vi "_LO_PAMP_set.vi"(9 "PAV配列":cluster{"VD":dbl, "VG ":dbl, "文字列":string}[](array[cluster]) {"VG" min=0.0 max=2.5; "VD" min=0.0 max=2.5}, 11 "Bias_LO_equip":T1={"Node address"=19, "CAN Interface"="CAN0", "Cartridge band"=10, "Slave Node in"={"Address"=19, "Serial Number"=[16, 71, 55, 76, 1, 8, 0, -15]}, "ObjHandle out"=89653312, "POL"=0, "sb"=1, "GPIB_SM (SIS S,V)"="24", "GPIB_DMM (SIS I)"="22", "GPIB_SM (MAG I) "="25", "GPIB_SG(LO)"="19", "GPIB_PW (PAMP) "="6", "GPIB_TMP1(8ch)"="12", "GPIB_TMP2(2ch)  "="13", "WCA_avg"=10, "Rsen"=10.0, "BiasModule"=1, "LOModule "=1, "WCA_LO_FREQ_SET"={"YTO Low freq. [GHz]"=14.42, "YTO High freq. [GHz]"=17.7, "Kvco"=1, "Lock Pol."=0, "SET LO FREQ"=72.5, "Multiplier"=6.0, "YTO (HEX)"=0, "YTO coarse( FREQ)"=25.0, "NULL PLL INTEGRATOR"=FALSE}, "Res for"=0} {"Res for" items=["none", "series res", "parallel res"]; "WCA_LO_FREQ_SET"."YTO coarse( FREQ)" min=25 max=150 step=0.0001 format="%.3f"; "WCA_LO_FREQ_SET"."Multiplier" min=3 max=6 step=3; "WCA_LO_FREQ_SET"."SET LO FREQ" min=25 max=150 step=0.0001 format="%.3f"; "WCA_LO_FREQ_SET"."Lock Pol." items=["Lower", "Upper"]; "WCA_LO_FREQ_SET"."Kvco" items=["7.5MHz/V", "15MHz/V"]; "WCA_LO_FREQ_SET"."YTO High freq. [GHz]" format="%.3f"; "WCA_LO_FREQ_SET"."YTO Low freq. [GHz]" format="%.3f"; "LOModule" items=["Manual Gunn+PAMP", "B10Lab LO", "WCA LO", "", "YIG発信器"]; "BiasModule" items=["B10Lab Bias", "WCA BiasModule"]; "Slave Node in"."Serial Number" format="%.0x"; "Slave Node in"."Address" format="%.0x"; "Cartridge band" max=10 step=1; "Node address" format="%.0x"}) -> ()   [LabVIEW 2017]
panel:
  in  "WCA_PA_SET":T2={"PA_A_DRAIN_V"=1.0, "PA_A_GATE_V"=0.0, "PA_B_DRAIN_V"=0.0, "PA_B_GATE_V"=0.0} {"PA_B_DRAIN_V" min=0.0 max=2.5; "PA_A_DRAIN_V" min=0.0 max=2.5}
  # "LO freq. [GHz]"
  # "YTO LOW\n/High Freq."
  # "ZERO Intgrtr"
  # "Node Address"
  # "Serial Number"
  # "Drain V"
  # "Gate V"
  # "PA_A (Pol1)"
  # "PA_B (Pol0)"
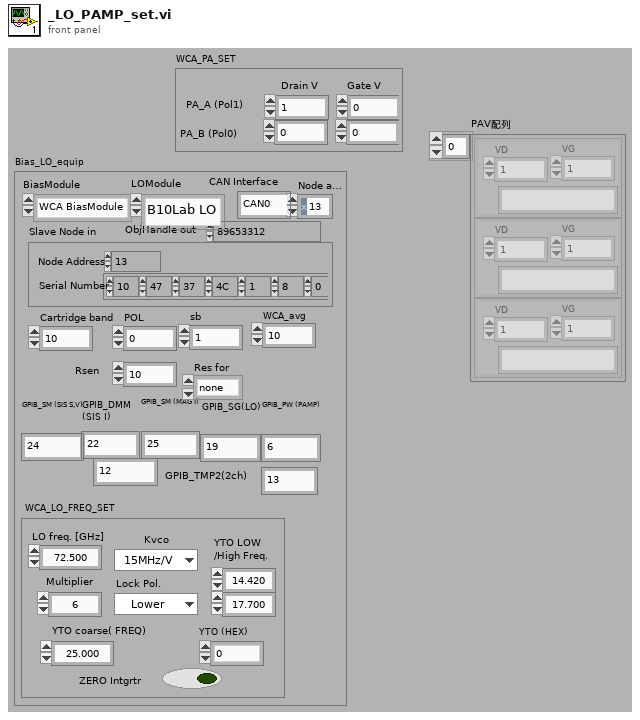
[diagram p1: front panel]
types:
  T1 = cluster{"Node address":u16, "CAN Interface":string, "Cartridge band":u32, "Slave Node in":cluster{"Address":i16, "Serial Number":i8[]}, "ObjHandle out":u32, "POL":u32, "sb":u32, "GPIB_SM (SIS S,V)":string, "GPIB_DMM (SIS I)":string, "GPIB_SM (MAG I) ":string, "GPIB_SG(LO)":string, "GPIB_PW (PAMP) ":string, "GPIB_TMP1(8ch)":string, "GPIB_TMP2(2ch)  ":string, "WCA_avg":i32, "Rsen":dbl, "BiasModule":u16, "LOModule ":u16, "WCA_LO_FREQ_SET":cluster{"YTO Low freq. [GHz]":sgl, "YTO High freq. [GHz]":sgl, "Kvco":u16, "Lock Pol.":u16, "SET LO FREQ":sgl, "Multiplier":sgl, "YTO (HEX)":u16, "YTO coarse( FREQ)":sgl, "NULL PLL INTEGRATOR":bool}, "Res for":u16}
  T2 = cluster{"PA_A_DRAIN_V":dbl, "PA_A_GATE_V":dbl, "PA_B_DRAIN_V":dbl, "PA_B_GATE_V":dbl}
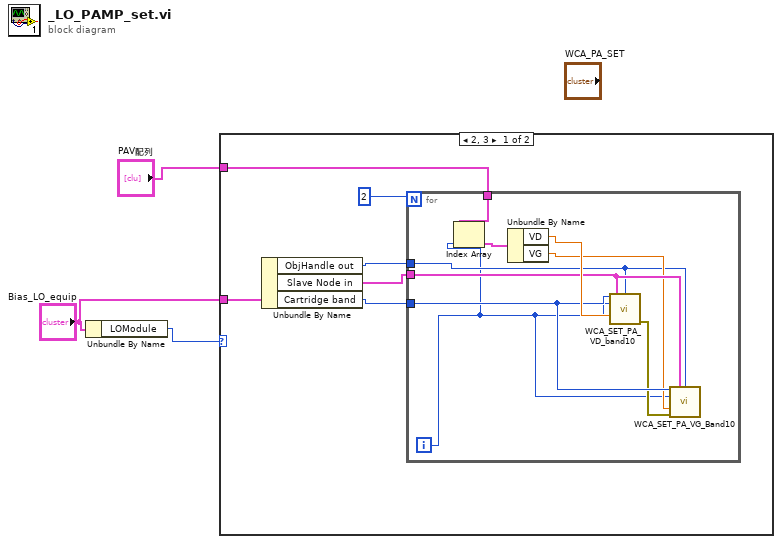
[diagram p0: block diagram]
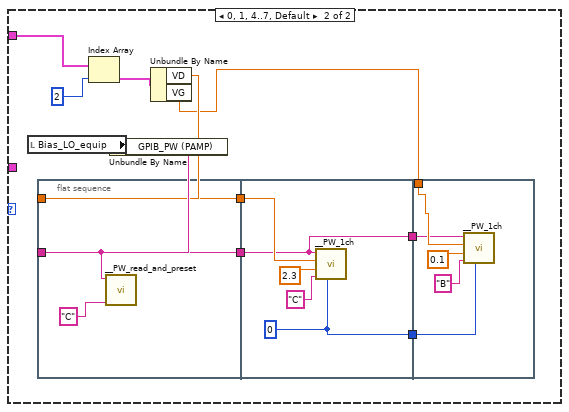
[diagram p2: hidden frame]
diagram:
  n1 = Unbundle By Name("Bias_LO_equip") -> ("LOModule"=w3:u16)
  n2 = case shown="2, 3" w3 {
    tunnel: "PAV配列" -> [w9 w29]
    tunnel: "Bias_LO_equip" -> [w8 _]
    frame 2, 3 {
      n3 = Unbundle By Name(w8) -> ("ObjHandle out"=w5:u32, "Slave Node in"=w7:cluster{"Address":i16, "Serial Number":i8[]}, "Cartridge band"=w6:u32)
      n4 = for {
        N: 2 -> [_]
        tunnel: w9 -> [w17]
        tunnel: w7 -> [w15]
        tunnel: w6 -> [w14]
        tunnel: w5 -> [w12]
        i -> [w10]
        n5 = Index Array(array=w17, index=w10) -> (element=w18:cluster{"VD":dbl, "VG ":dbl, "文字列":string})
        n6 = Unbundle By Name(w18) -> ("VD"=w16:dbl, "VG"=w13:dbl)
        n7 = call "WCA_SET_PA_VD_band10.vi"("Cartridge Band"=w14, "Slave Node in"=w15, "ObjHandle in"=w12, "POL（P0、P1）"=w10, "SET_PA_VD"=w16) -> ("error out"=w11:errorcluster)  [unwired: 9 in, 1 out]
        n8 = call "WCA_SET_PA_VG_Band10.vi"("Cartridge Band"=w14, "Slave Node in"=w15, "ObjHandle in"=w12, "POL（P0、P1）"=w10, "SET_PA_VG"=w13, "error in (no error)"=w11) -> ()  [unwired: 8 in, 2 out]
      }
    }
    frame 0, 1, 4..7, Default {
      n9 = local read "Bias_LO_equip"() -> (w26:T1)
      n10 = flat-sequence {
        tunnel: w24 -> [w32]
        tunnel: w25 -> [w31]
        tunnel: [w31] -> w21
        tunnel: [w32] -> w20
        tunnel: [w34] -> w22
        tunnel: w21 -> [w34]
        tunnel: w20 -> [w35]
        tunnel: [w33] -> w19
        tunnel: w23 -> [w40]
        tunnel: w22 -> [w39]
        tunnel: w19 -> [w38]
        frame #0 {
          n11 = call "__PW_read_and_preset.vi"("MAXCh（A,B,C,D）"="C", "GPIB"=w31) -> ()  [unwired: 10 in]
        }
        frame #1 {
          w33 = 0
          n12 = call "__PW_1ch.vi"("Wait(ms)"=w33, "Ch（A,B,C,D）"="C", "A(A)"=2.3, "V(V)"=w35, "GPIB"=w34) -> ()  [unwired: 5 in, 2 out]
        }
        frame #2 {
          n13 = call "__PW_1ch.vi"("Wait(ms)"=w38, "Ch（A,B,C,D）"="B", "A(A)"=0.1, "V(V)"=w40, "GPIB"=w39) -> ()  [unwired: 5 in, 2 out]
        }
      }
      n14 = Index Array(array=w29, index=2) -> (element=w27:cluster{"VD":dbl, "VG ":dbl, "文字列":string})
      n15 = Unbundle By Name(w26) -> ("GPIB_PW (PAMP)"=w25:string)
      n16 = Unbundle By Name(w27) -> ("VD"=w24:dbl, "VG"=w23:dbl)
    }
  }
